vi "Auto-Approach.vi"() -> ()   [LabVIEW 2016]
doc: "Programming Interface Example: Automatic approach implemented using Nanonis Programming Interface functions. This can be used if you want to execute special functions after each motor step or if you want to control your motor directly from LabVIEW.\n\n- Nanonis Programming Interface -"
uses:
  Nanonis Prog Interface.lvlib
panel:
  out "Surface reached":bool
  in  "Wait for motor (ms)":u32=1000
  in  "Motor steps":u16=1
  in  "stop":bool
  # "Example for the Nanonis SPM Control software \nprogramming interface (see diagram)"
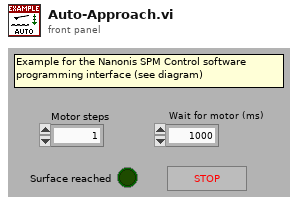
[diagram p1: front panel]
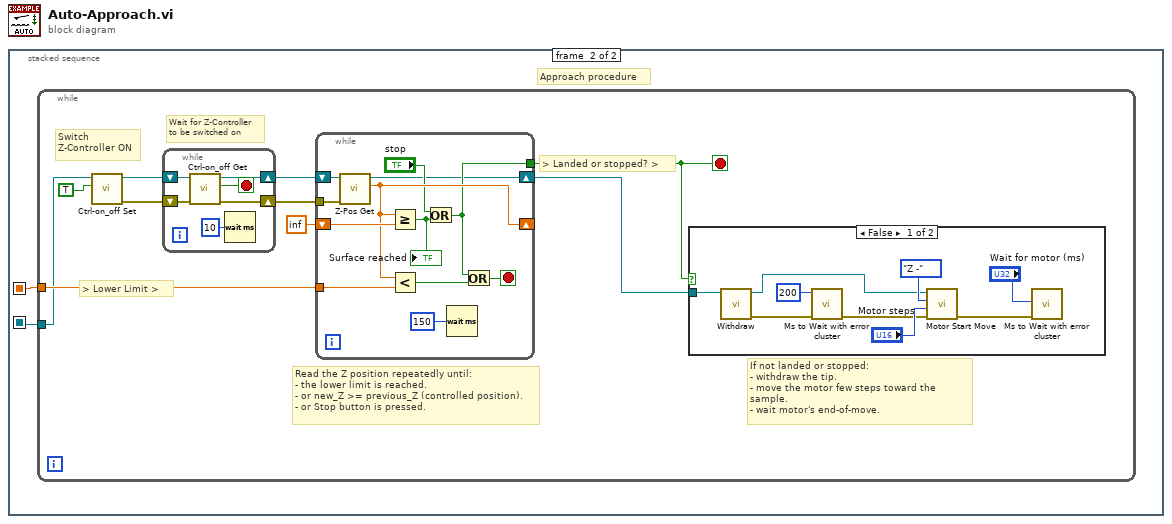
[diagram p0: block diagram]
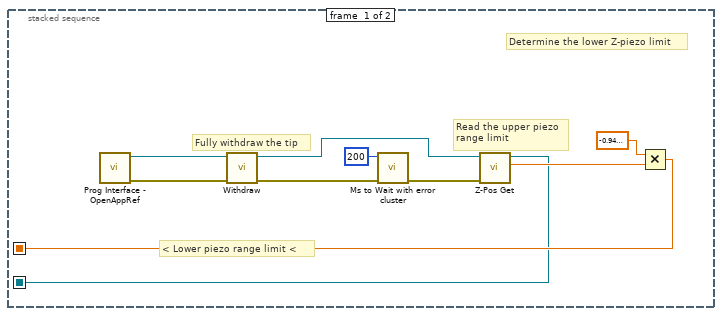
[diagram p2: hidden frame]
diagram:
  n1 = stacked-sequence {
    seq-local: [w9 _] -> [_ w12]
    seq-local: [w2 _] -> [_ w11]
    frame #0 {
      # "Read the upper piezo\nrange limit"
      # "Fully withdraw the tip"
      # "< Lower piezo range limit <"
      # "Determine the lower Z-piezo limit"
      n2 = call <userlib>:"Prog Interface - OpenAppRef.vi"() -> ("Error out"=w8:errorcluster, "Application reference"=w3:refnum<vi>)  [unwired: 6 in]
      n3 = call <userlib>:"Withdraw.vi"("Error in (no error)"=w8, "Application ref in"=w3) -> ("Error out"=w5:errorcluster, "Application ref out"=w1:refnum<vi>)  [unwired: 8 in]
      n4 = call "Ms to Wait with error cluster.vi"("error in (no error)"=w5, "milliseconds to wait"=u32 200) -> ("error out"=w4:errorcluster)  [unwired: 4 in, 1 out]
      n5 = call <userlib>:"Z-Pos Get.vi"("error in (no error)"=w4, "Application ref in"=w1) -> ("Z position (m)"=w7:sgl, "Application ref out"=w2:refnum<vi>)  [unwired: 7 in, 1 out]
      n6 = Multiply(x=sgl -0.95, y=w7) -> (x*y=w9:sgl)
    }
    frame #1 {
      # "Approach procedure"
      n7 = while {
        tunnel: w12 -> [w21]
        tunnel: w11 -> [w16]
        stop <- w22 stop-if-true
        # "Wait for Z-Controller\nto be switched on"
        # "> Lower Limit >"
        # "Switch Z-Controller ON"
        # "> Landed or stopped? >"
        # "Read the Z position repeatedly until:\n- the lower limit is reached.\n- or new_Z >= previous_Z (controlled position).\n- or Stop button is pressed."
        # "If not landed or stopped:\n- withdraw the tip.\n- move the motor few steps toward the sample.\n- wait motor's end-of-move."
        n8 = call <userlib>:"Ctrl-on_off Set.vi"("Z Controller ON/OFF"=TRUE ("Ctrl on/off"), "Application ref in"=w16) -> ("error out"=w18:errorcluster, "Application ref out"=w15:refnum<vi>)  [unwired: 8 in]
        n9 = while {
          shift-right: [w28] -> w17
          shift-left: w18 -> [w27]
          shift-right: [w23] -> w14
          shift-left: w15 -> [w24]
          stop <- w26 stop-if-true
          n10 = call <userlib>:"Ctrl-on_off Get.vi"("error in (no error)"=w27, "Application ref in"=w24) -> ("error out"=w28:errorcluster, "Z-Controller on/off status"=w26:bool, "Application ref out"=w23:refnum<vi>)  [unwired: 7 in]
          n11 = Wait (ms)(milliseconds to wait=u32 10) -> ()  [unwired: 1 out]
        }
        n12 = while {
          shift-right: [w38] -> _
          shift-left: sgl inf ("Z-pos (m)") -> [w40]
          tunnel: [w34] -> w22
          tunnel: w21 -> [w32]
          tunnel: w17 -> [w31]
          shift-right: [w29] -> w13
          shift-left: w14 -> [w30]
          stop <- w35 stop-if-true
          n13 = call <userlib>:"Z-Pos Get.vi"("error in (no error)"=w31, "Application ref in"=w30) -> ("Z position (m)"=w38:sgl, "Application ref out"=w29:refnum<vi>)  [unwired: 7 in, 1 out]
          n14 = Greater Or Equal?(x=w38, y=w40) -> (x >= y?=w37:bool)
          "Surface reached" <- w37
          n15 = Less?(x=w38, y=w32) -> (x < y?=w36:bool)
          n16 = Or(x="stop", y=w37) -> (x .or. y?=w34:bool)
          n17 = Wait (ms)(milliseconds to wait=u32 150) -> ()  [unwired: 1 out]
          n18 = Or(x=w34, y=w36) -> (x .or. y?=w35:bool)
        }
        n19 = case shown="False" w22 {
          tunnel: w13 -> [w42 _]
          frame False {
            n20 = call <userlib>:"Withdraw.vi"("Application ref in"=w42) -> ("Error out"=w47:errorcluster, "Application ref out"=w41:refnum<vi>)  [unwired: 9 in]
            n21 = call "Ms to Wait with error cluster.vi"("error in (no error)"=w47, "milliseconds to wait"=u32 200) -> ("error out"=w46:errorcluster)  [unwired: 4 in, 1 out]
            n22 = call <userlib>:"Motor Start Move.vi"("Error in (no error)"=w46, "Number of steps"="Motor steps", "Direction"=enum16{"X +", "X -", "Y +", "Y -", "Z +", "Z -"}."Z -", "Application ref in"=w41) -> ("Error out"=w44:errorcluster)  [unwired: 5 in, 1 out]
            n23 = call "Ms to Wait with error cluster.vi"("error in (no error)"=w44, "milliseconds to wait"="Wait for motor (ms)") -> ()  [unwired: 4 in, 2 out]
          }
          frame True {
          }
        }
      }
    }
  }
